vi "UpdateCANData.vi"() -> ()   [LabVIEW 2011]
uses:
  _USB_CAN_T_R_Unit_.ctl
  <vilib>/Utility/file.llb/Write To Spreadsheet File (string).vi
panel:
  in  "sPth_Sel":bool
  out "sv_pth":path
  in  "TSFormat":enum16{"原始值", "实际值"}(ring)
  in  "check2":bool
  in  "rate3":refnum<vi>
  in  "rate2":refnum<vi>
  in  "rate1":refnum<vi>
  in  "errcnt2":refnum<vi>
  in  "Trate2":bool
  in  "Trate1":bool
  in  "Rrate2":bool
  in  "Rrate1":bool
  in  "ForceUpt":bool
  in  "format":enum16{"hex", "dec", "oct", "bin"}(ring)
  in  "ID合并":bool
  in  "SaveCnt":refnum<vi>
  in  "path":refnum<vi>
  in  "rate0":refnum<vi>
  in  "vi ref":refnum<vi>
  in  "highspd":bool
  in  "cancelEvt":refnum<user-event>
  in  "check1":bool
  in  "errcnt1":refnum<vi>
  in  "save":bool
  in  "disp":bool=TRUE
  in  "stop":bool
  in  "savefile":bool
  in  "UseFilter":bool
  in  "Filter":u32[](array[numeric])
  in  "clear":bool
  in  "Enable":bool
  in  "list ref":refnum<vi>
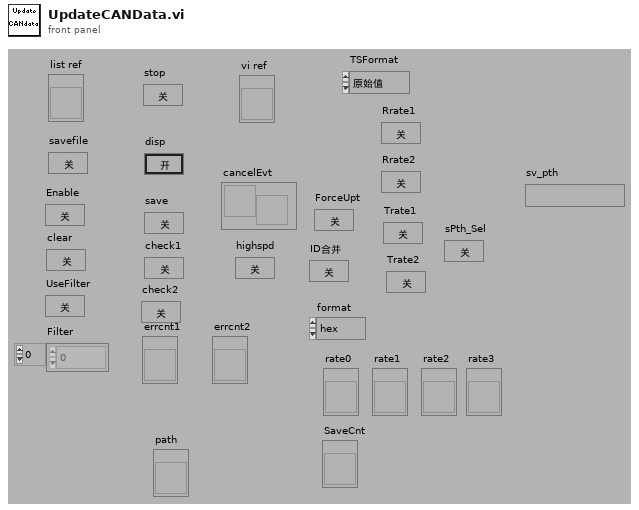
[diagram p1: front panel]
types:
  T1 = typedef "_USB_CAN_T_R_Unit_.ctl" = cluster{"time":timestamp, "channel":u16, "TimeStamp":u32, "tr":enum16{"接收", "发送"}, "id":u32, "Type":enum16{"数据帧", "远程帧"}, "Format":enum16{"标准帧", "扩展帧"}, "len":u8, "data":u8[]}
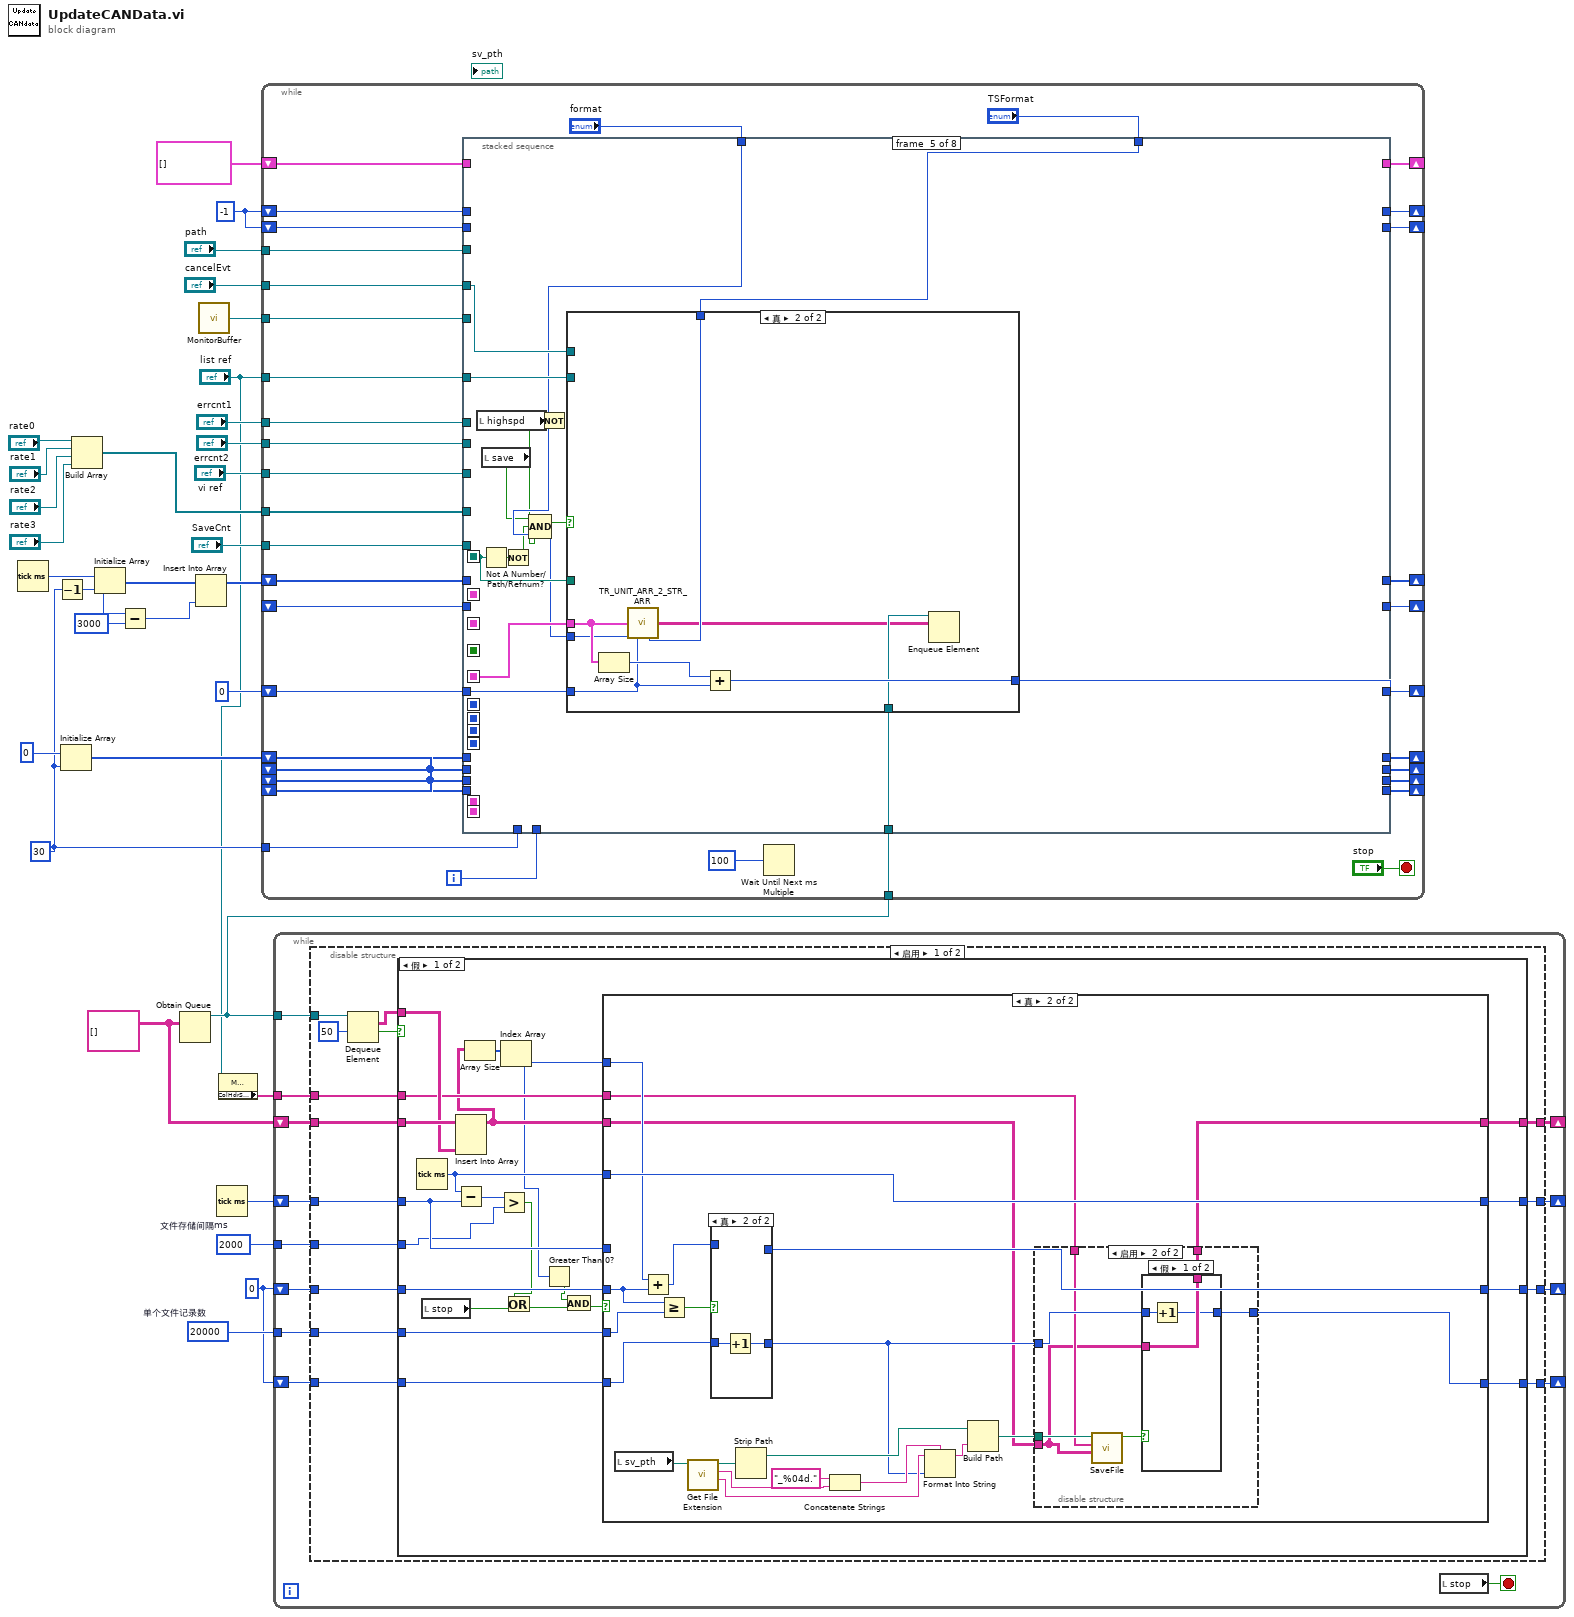
[diagram p0: block diagram]
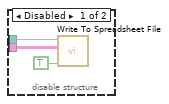
[diagram p3: hidden frame]
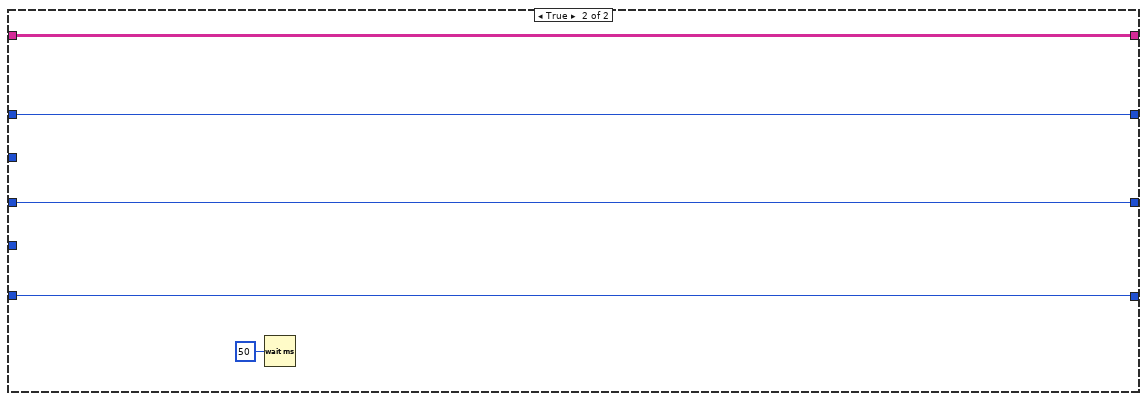
[diagram p6: hidden frame]
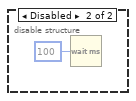
[diagram p7: hidden frame]
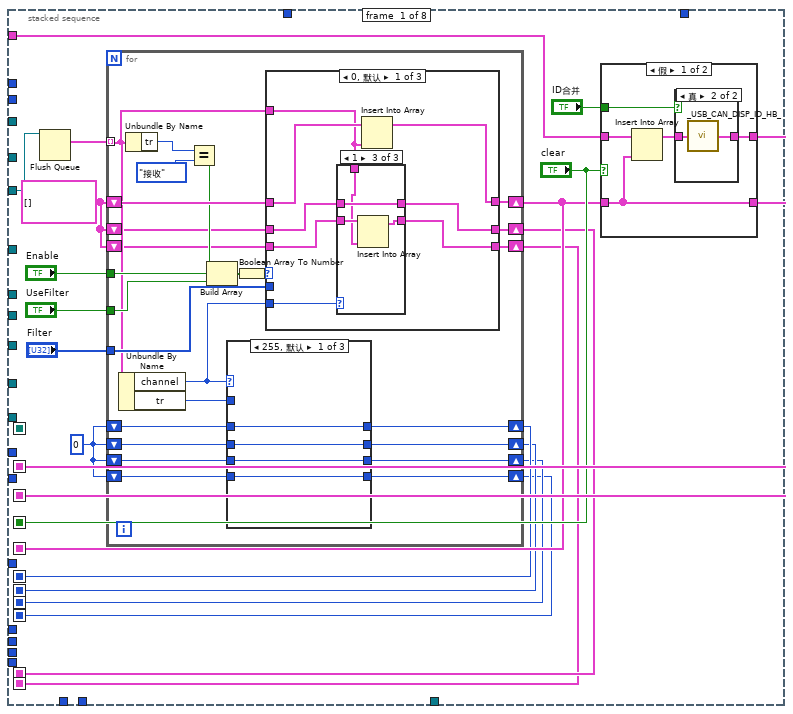
[diagram p8: hidden frame]
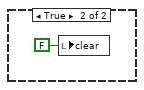
[diagram p10: hidden frame]
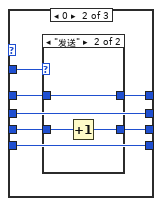
[diagram p11: hidden frame]
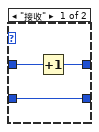
[diagram p12: hidden frame]
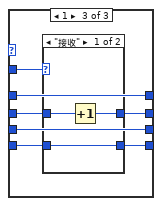
[diagram p13: hidden frame]
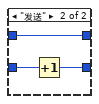
[diagram p14: hidden frame]
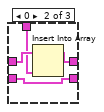
[diagram p16: hidden frame]
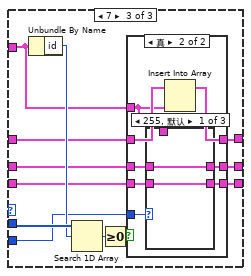
[diagram p18: hidden frame]
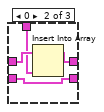
[diagram p20: hidden frame]
diagram:
  w2 = u32 2000  # 文件存储间隔ms
  w3 = 20000  # 单个文件记录数
  w1 = 0
  w8 = string[][] [] ("strTable")
  w25 = 30 ("维数大小")
  w6 = i64 -1 ("U64")
  n1 = Tick Count (ms)() -> (millisecond timer value=w11:u32)
  n2 = Decrement(x=w25) -> (x-1=w24:i32)
  n3 = Initialize Array(0, w25) -> (w17:i32[])
  n4 = Build Array("rate0", "rate1", "rate2", "rate3") -> (w12:refnum<vi>[])
  n5 = Initialize Array(w11, w24) -> (w23:u32[])
  n6 = Subtract(x=w11, y=u32 3000) -> (x-y=w20:u32)
  n7 = Obtain Queue(element data type=w8) -> (queue out=w9:refnum<queue>)  [unwired: 4 in, 2 out]
  n8 = Insert Into Array(array=w23, new element=w20) -> (w22:u32[])  [unwired: 1 in]
  n9 = call "MonitorBuffer.vi"() -> ("USB_CAN_M_BUF"=w32:refnum<queue>)  [unwired: 1 in]
  n10 = Tick Count (ms)() -> (millisecond timer value=w4:u32)
  n11 = property class="MCListbox (严格)"(reference="list ref") -> ("ColHdrString"=w5:string[])  [unwired: 1 in, 2 out]
  n12 = while {
    tunnel: w32 -> [w67]
    shift-right: [w65] -> _
    shift-left: T1[] [] -> [w66]
    tunnel: "list ref" -> [w64]
    shift-right: [w61] -> _
    shift-left: w6 -> [w63]
    tunnel: "errcnt1" -> [w62]
    tunnel: "cancelEvt" -> [w60]
    shift-right: [w58] -> _
    shift-left: 0 -> [w59]
    tunnel: "vi ref" -> [w57]
    shift-right: [w55] -> _
    shift-left: w17 -> [w56]
    tunnel: w25 -> [w53]
    tunnel: w12 -> [w52]
    shift-right: [w50] -> _
    shift-left: w22 -> [w51]
    tunnel: "SaveCnt" -> [w48]
    tunnel: "errcnt2" -> [w46]
    shift-right: [w42] -> _
    shift-left: w17 -> [w45]
    shift-right: [w41] -> _
    shift-left: w17 -> [w44]
    shift-right: [w40] -> _
    shift-left: w17 -> [w43]
    shift-right: [w38] -> _
    shift-left: w6 -> [w39]
    shift-right: [w36] -> _
    shift-left: _ -> [w37]
    tunnel: "path" -> [w34]
    tunnel: w9 -> [w33]
    i -> [w54]
    stop <- "stop" stop-if-true
    n13 = stacked-sequence {
      seq-local: [w85 _ _ _ _ _ _ _] -> [_ _ w300 _ _ w419 _ _]
      seq-local: [w84 _ _ _ _ _ _ _] -> [_ _ w297 _ _ _ _ _]
      seq-local: [_ _ _ w357 _ _ _ _] -> [_ _ _ _ w399 _ _ _]
      seq-local: ["clear" _ _ _ _ _ _ _] -> [_ _ w294 _ _ _ _ _]
      seq-local: [w82 _ _ _ _ _ _ _] -> [_ _ _ _ w396 _ _ _]
      seq-local: [w81 _ _ _ _ _ _ _] -> [_ w228 w292 _ _ _ _ _]
      seq-local: [w80 _ _ _ _ _ _ _] -> [_ w220 w291 _ _ _ _ _]
      seq-local: [w79 _ _ _ _ _ _ _] -> [_ w219 w290 _ _ _ _ _]
      seq-local: [w78 _ _ _ _ _ _ _] -> [_ w218 w289 _ _ _ _ _]
      seq-local: [w77 _ _ _ _ _ _ _] -> [_ _ _ _ _ _ w452 _]
      seq-local: [w76 _ _ _ _ _ _ _] -> [_ _ _ _ _ _ _ w508]
      tunnel: w67 -> [w87 _ _ _ _ _ _ _]
      tunnel: w66 -> [w86 _ _ _ _ _ w455 _]
      tunnel: [_ _ w300 _ _ _ _ _] -> w65
      tunnel: w64 -> [_ _ w299 _ w398 w418 _ _]
      tunnel: w63 -> [_ _ _ _ _ _ w457 _]
      tunnel: w62 -> [_ _ w286 _ _ _ w450 _]
      tunnel: [_ _ _ _ _ _ w458 _] -> w61
      tunnel: w60 -> [_ _ _ _ w397 _ _ _]
      tunnel: w59 -> [_ _ _ _ w395 _ _ _]
      tunnel: [_ _ _ _ w394 _ _ _] -> w58
      tunnel: w57 -> [_ _ w298 _ _ _ _ _]
      tunnel: w56 -> [_ w229 _ _ _ _ _ _]
      tunnel: [_ w227 _ _ _ _ _ _] -> w55
      tunnel: w54 -> [_ w224 _ _ _ _ _ _]
      tunnel: w53 -> [_ w230 _ _ _ _ _ _]
      tunnel: w52 -> [_ w214 _ _ _ _ _ _]
      tunnel: w51 -> [_ w226 _ _ _ _ _ _]
      tunnel: [_ w225 _ _ _ _ _ _] -> w50
      tunnel: w34 -> [_ _ _ w363 _ _ _ _]
      tunnel: w48 -> [_ _ w287 _ _ w417 _ _]
      tunnel: "format" -> [_ _ w296 _ w393 w416 _ _]
      tunnel: w46 -> [_ _ w285 _ _ _ _ w507]
      tunnel: w45 -> [_ w223 _ _ _ _ _ _]
      tunnel: w44 -> [_ w222 _ _ _ _ _ _]
      tunnel: w43 -> [_ w221 _ _ _ _ _ _]
      tunnel: [_ w217 _ _ _ _ _ _] -> w42
      tunnel: [_ w216 _ _ _ _ _ _] -> w41
      tunnel: [_ w215 _ _ _ _ _ _] -> w40
      tunnel: w39 -> [_ _ _ _ _ _ _ w510]
      tunnel: [_ _ _ _ _ _ _ w511] -> w38
      tunnel: w37 -> [_ _ w293 _ _ _ _ _]
      tunnel: [_ _ w295 _ _ _ _ _] -> w36
      tunnel: "TSFormat" -> [_ _ w288 _ w392 _ _ _]
      tunnel: w33 -> [_ _ _ _ w391 _ _ _]
      frame #0 {
        w70 = 0 ("和")
        w69 = T1[] []
        n14 = Flush Queue(queue=w87) -> (remaining elements=w72:T1[])  [unwired: 1 in, 2 out]
        n15 = for {
          tunnel: w72 -> [w111] mode=indexing
          shift-right: [w113] -> w82
          shift-left: w69 -> [w115]
          tunnel: "Enable" -> [w119]
          tunnel: "UseFilter" -> [w118]
          tunnel: "Filter" -> [w114]
          shift-right: [w105] -> w81
          shift-left: w70 -> [w109]
          shift-right: [w104] -> w80
          shift-left: w70 -> [w108]
          shift-right: [w103] -> w79
          shift-left: w70 -> [w107]
          shift-right: [w102] -> w78
          shift-left: w70 -> [w106]
          shift-right: [w99] -> w77
          shift-left: w69 -> [w101]
          shift-right: [w98] -> w76
          shift-left: w69 -> [w100]
          n16 = Unbundle By Name(w111) -> ("channel"=w97:u16, "tr"=w110:enum16{"接收", "发送"})
          n17 = Unbundle By Name(w111) -> ("tr"=w121:enum16{"接收", "发送"})
          n18 = Equal?(x=w121, y=enum16{"接收", "发送"}."接收") -> (x = y?=w112:bool)
          n19 = Build Array(w112, w119, w118) -> (w117:bool[])
          n20 = case shown="255, 默认" w97 {
            tunnel: w110 -> [_ w132 w145]
            tunnel: w109 -> [w125 w130 w144]
            tunnel: w108 -> [w124 w127 w142]
            tunnel: w107 -> [w123 w128 w143]
            tunnel: w106 -> [w122 w131 w141]
            tunnel: [w125 w129 w144] -> w105
            tunnel: [w124 w127 w139] -> w104
            tunnel: [w123 w126 w143] -> w103
            tunnel: [w122 w131 w140] -> w102
            frame 255, Default {
            }
            frame 0 {
              n21 = case shown="\"发送\"" w132 {
                tunnel: w130 -> [w135 w138]
                tunnel: [w134 w138] -> w129
                tunnel: w128 -> [w133 w137]
                tunnel: [w133 w136] -> w126
                frame "接收" {
                  n22 = Increment(x=w135) -> (x+1=w134:i32)
                }
                frame "发送" {
                  n23 = Increment(x=w137) -> (x+1=w136:i32)
                }
              }
            }
            frame 1 {
              n24 = case shown="\"接收\"" w145 {
                tunnel: w142 -> [w148 w149]
                tunnel: w141 -> [w146 w151]
                tunnel: [w146 w150] -> w140
                tunnel: [w147 w149] -> w139
                frame "接收" {
                  n25 = Increment(x=w148) -> (x+1=w147:i32)
                }
                frame "发送" {
                  n26 = Increment(x=w151) -> (x+1=w150:i32)
                }
              }
            }
          }
          n27 = Boolean Array To Number(Boolean array=w117) -> (number=w116:u32)
          n28 = case shown="0, 默认" w116 {
            tunnel: w115 -> [w158 w172 w180]
            tunnel: w111 -> [w157 _ w179]
            tunnel: w114 -> [_ _ w184]
            tunnel: [w159 w172 w178] -> w113
            tunnel: w101 -> [w155 w171 w176]
            tunnel: w100 -> [w154 w170 w175]
            tunnel: [w153 w171 w174] -> w99
            tunnel: [w152 w170 w173] -> w98
            tunnel: w97 -> [w156 _ w177]
            frame 0, Default {
              n29 = case shown="1" w156 {
                tunnel: w155 -> [w161 w165 w169]
                tunnel: w154 -> [w160 w163 w167]
                tunnel: [w161 w164 w169] -> w153
                tunnel: [w160 w163 w168] -> w152
                tunnel: w157 -> [_ w162 w166]
                frame 255, Default {
                }
                frame 0 {
                  n30 = Insert Into Array(array=w165, new element=w162) -> (w164:T1[])  [unwired: 1 in]
                }
                frame 1 {
                  n31 = Insert Into Array(array=w167, new element=w166) -> (w168:T1[])  [unwired: 1 in]
                }
              }
              n32 = Insert Into Array(array=w158, new element=w157) -> (w159:T1[])  [unwired: 1 in]
            }
            frame 1, 5 {
            }
            frame 7 {
              n33 = Unbundle By Name(w179) -> ("id"=w183:u32)
              n34 = Search 1D Array(1D array=w184, element=w183) -> (index of element=w182:i32)  [unwired: 1 in]
              n35 = Greater Or Equal To 0?(x=w182) -> (x >= 0?=w181:bool)
              n36 = case shown="真" w181 {
                tunnel: w180 -> [w187 w195]
                tunnel: w179 -> [_ w188]
                tunnel: [w187 w194] -> w178
                tunnel: w177 -> [_ w193]
                tunnel: w176 -> [w186 w192]
                tunnel: w175 -> [w185 w191]
                tunnel: [w186 w190] -> w174
                tunnel: [w185 w189] -> w173
                frame False {
                }
                frame True {
                  n37 = case shown="255, 默认" w193 {
                    tunnel: w192 -> [w197 w201 w205]
                    tunnel: w191 -> [w196 w199 w203]
                    tunnel: [w197 w200 w205] -> w190
                    tunnel: [w196 w199 w204] -> w189
                    tunnel: w188 -> [_ w198 w202]
                    frame 255, Default {
                    }
                    frame 0 {
                      n38 = Insert Into Array(array=w201, new element=w198) -> (w200:T1[])  [unwired: 1 in]
                    }
                    frame 1 {
                      n39 = Insert Into Array(array=w203, new element=w202) -> (w204:T1[])  [unwired: 1 in]
                    }
                  }
                  n40 = Insert Into Array(array=w195, new element=w188) -> (w194:T1[])  [unwired: 1 in]
                }
              }
            }
          }
        }
        n41 = case shown="假" "clear" {
          tunnel: w82 -> [w92 _]
          tunnel: w86 -> [w91 _]
          tunnel: [w88 _] -> w85
          tunnel: [w92 _] -> w84
          tunnel: "ID合并" -> [w90 _]
          frame False {
            n42 = Insert Into Array(array=w91, new element=w92) -> (w89:T1[])  [unwired: 1 in]
            n43 = case shown="真" w90 {
              tunnel: w89 -> [w93 w95]
              tunnel: [w93 w94] -> w88
              frame False {
              }
              frame True {
                n44 = call "_USB_CAN_DISP_ID_HB_.vi"("Arr In"=w95) -> ("Arr Out"=w94:T1[])
              }
            }
          }
          frame True {
            n45 = local write "clear"(FALSE ("clear")) -> ()
          }
        }
      }
      frame #1 {
        n46 = Tick Count (ms)() -> (millisecond timer value=w213:u32)
        n47 = Quotient & Remainder(x=w224, y=w230) -> (x-y*floor(x/y)=w210:i32)  [unwired: 1 out]
        n48 = Replace Array Subset(array=w229, new element=w228, index=w210) -> (w227:i32[])
        n49 = Replace Array Subset(array=w223, new element=w220, index=w210) -> (w217:i32[])
        n50 = Replace Array Subset(array=w222, new element=w219, index=w210) -> (w216:i32[])
        n51 = Replace Array Subset(array=w221, new element=w218, index=w210) -> (w215:i32[])
        n52 = Replace Array Subset(array=w226, new element=w213, index=w210) -> (w225:u32[])
        n53 = Quotient & Remainder(x=w224, y=5) -> (x-y*floor(x/y)=w211:i32)  [unwired: 1 out]
        n54 = case shown="0" w211 {
          tunnel: w227 -> [_ w248]
          tunnel: w225 -> [_ w245]
          tunnel: w217 -> [_ w238]
          tunnel: w216 -> [_ w237]
          tunnel: w215 -> [_ w236]
          tunnel: w214 -> [_ w244]
          tunnel: "Rrate1" -> [_ w234]
          tunnel: "Rrate2" -> [_ w233]
          tunnel: "Trate1" -> [_ w232]
          tunnel: "Trate2" -> [_ w231]
          frame -1, Default {
          }
          frame 0 {
            w235 = 1000.0 ("y")
            n55 = Array Max & Min(array=w245) -> (max value=w247:u32, min value=w246:u32)  [unwired: 2 out]
            n56 = Subtract(x=w247, y=w246) -> (x-y=w239:u32)
            n57 = Index Array(array=w244) -> (element #1=w243:refnum<vi>, element #2=w242:refnum<vi>, element #3=w241:refnum<vi>, element #4=w240:refnum<vi>)  [unwired: 4 in]
            n58 = case shown="真" w234 {
              tunnel: w248 -> [_ w276]
              tunnel: w243 -> [_ w272]
              tunnel: w239 -> [_ w271]
              tunnel: w235 -> [_ w270]
              frame False {
              }
              frame True {
                n59 = Add Array Elements(numeric array=w276) -> (sum=w275:i32)
                n60 = Divide(x=w275, y=w271) -> (x/y=w274:dbl)
                n61 = Multiply(x=w274, y=w270) -> (x*y=w273:dbl)
                n62 = property class="DigNum (严格)"(reference=w272, "Value"=w273) -> ()  [unwired: 1 in, 2 out]
              }
            }
            n63 = case shown="真" w233 {
              tunnel: w242 -> [_ w266]
              tunnel: w239 -> [_ w265]
              tunnel: w238 -> [_ w264]
              tunnel: w235 -> [_ w263]
              frame False {
              }
              frame True {
                n64 = Add Array Elements(numeric array=w264) -> (sum=w267:i32)
                n65 = Divide(x=w267, y=w265) -> (x/y=w268:dbl)
                n66 = Multiply(x=w268, y=w263) -> (x*y=w269:dbl)
                n67 = property class="DigNum (严格)"(reference=w266, "Value"=w269) -> ()  [unwired: 1 in, 2 out]
              }
            }
            n68 = case shown="真" w232 {
              tunnel: w241 -> [_ w259]
              tunnel: w239 -> [_ w258]
              tunnel: w237 -> [_ w257]
              tunnel: w235 -> [_ w256]
              frame False {
              }
              frame True {
                n69 = Add Array Elements(numeric array=w257) -> (sum=w262:i32)
                n70 = Divide(x=w262, y=w258) -> (x/y=w261:dbl)
                n71 = Multiply(x=w261, y=w256) -> (x*y=w260:dbl)
                n72 = property class="DigNum (严格)"(reference=w259, "Value"=w260) -> ()  [unwired: 1 in, 2 out]
              }
            }
            n73 = case shown="真" w231 {
              tunnel: w240 -> [_ w252]
              tunnel: w239 -> [_ w251]
              tunnel: w236 -> [_ w250]
              tunnel: w235 -> [_ w249]
              frame False {
              }
              frame True {
                n74 = Add Array Elements(numeric array=w250) -> (sum=w253:i32)
                n75 = Divide(x=w253, y=w251) -> (x/y=w254:dbl)
                n76 = Multiply(x=w254, y=w249) -> (x*y=w255:dbl)
                n77 = property class="DigNum (严格)"(reference=w252, "Value"=w255) -> ()  [unwired: 1 in, 2 out]
              }
            }
          }
        }
      }
      frame #2 {
        n78 = Not A Number/Path/Refnum?(number/path/refnum=w299) -> (NaN/Path/Refnum?=w284:bool)
        n79 = Empty Array?(array=w297) -> (empty?=w282:bool)
        n80 = Compound Arithmetic op=AND("disp", invert w284, invert w282, invert "highspd") -> (w281:bool)
        n81 = Compound Arithmetic op=ADD(w292, w291, w290, w289) -> (w278:i32)
        n82 = Compound Arithmetic op=OR("ForceUpt", w281, w294) -> (w280:bool)
        n83 = case shown="真" w280 {
          tunnel: w299 -> [_ w321]
          tunnel: w300 -> [_ w322]
          tunnel: w298 -> [_ w320]
          tunnel: w297 -> [_ w319]
          tunnel: w296 -> [_ w318]
          tunnel: w293 -> [w301 w307]
          tunnel: [w301 w317] -> w295
          tunnel: "ForceUpt" -> [_ w316]
          tunnel: w294 -> [_ w315]
          tunnel: w278 -> [_ w313]
          tunnel: w288 -> [_ w305]
          tunnel: w287 -> [_ _]
          tunnel: w286 -> [_ w303]
          tunnel: w285 -> [_ w302]
          frame False {
          }
          frame True {
            n84 = Tick Count (ms)() -> (millisecond timer value=w314:u32)
            n85 = Greater?(x=w313, y=0) -> (0:w306:bool)
            n86 = Subtract(x=w314, y=w307) -> (x-y=w311:u32)
            n87 = Greater?(x=w311, y=u32 300) -> (0:w309:bool)
            n88 = And(x=w309, y=w306) -> (x .and. y?=w308:bool)
            n89 = Compound Arithmetic op=OR(w316, w315, w308, w306) -> (w304:bool)
            n90 = case shown="真" w304 {
              tunnel: w322 -> [_ w332]
              tunnel: w321 -> [_ w331]
              tunnel: w320 -> [_ w330]
              tunnel: w319 -> [_ w329]
              tunnel: w318 -> [_ w328]
              tunnel: [w323 w327] -> w317
              tunnel: w314 -> [_ w327]
              tunnel: w307 -> [w323 _]
              tunnel: w305 -> [_ w326]
              tunnel: w303 -> [_ w325]
              tunnel: w302 -> [_ w324]
              frame False {
              }
              frame True {
                n91 = stacked-sequence {
                  tunnel: w332 -> [_ w349 _]
                  tunnel: w331 -> [_ w351 _]
                  tunnel: w330 -> [w333 _ w352]
                  tunnel: w329 -> [_ _ _]
                  tunnel: w328 -> [_ w350 _]
                  tunnel: w326 -> [_ w341 _]
                  tunnel: w325 -> [_ _ _]
                  tunnel: w324 -> [_ _ _]
                  frame #0 {
                    n92 = property class="VI"(reference=w333) -> (error out=w334:errorcluster, "Panel"=w336:refnum<vi>)  [unwired: 1 in, 1 out]
                    n93 = property class="Pnl"(reference=w336, error in=w334, "DeferPanUpdts"=TRUE ("延迟前面板更新")) -> ()  [unwired: 2 out]
                  }
                  frame #1 {
                    n94 = Array Size(array=w349) -> (size(s)=w347:i32)
                    n95 = Subtract(x=w347, y=200) -> (x-y=w343:i32)
                    n96 = Less Than 0?(x=w343) -> (x < 0?=w345:bool)
                    n97 = Select(t=0, s=w345, f=w343) -> (s? t:f=w342:i32)
                    n98 = Array Subset(array=w349, index=w342) -> (w348:T1[])  [unwired: 1 in]
                    n99 = call "TR_UNIT_ARR_2_STR_ARR.vi"("offset"=w342, "TR_Unit_Arr"=w348, "format"=w350, "TSFormat"=w341) -> ("smb"=w338:i32[], "strTable"=w339:string[][])  [unwired: 10 in]
                    n100 = property class="MCListbox (严格)"(reference=w351, "ItemNames"=w339, "ItemSyms"=w338) -> (reference out=w340:refnum<vi>)  [unwired: 1 in, 1 out]
                    n101 = call "DispLastRow(MList).vi"("显示尾行"=TRUE, "MCListbox引用句柄"=w340) -> ()  [unwired: 8 in, 2 out]
                  }
                  frame #2 {
                    n102 = property class="VI"(reference=w352) -> (error out=w353:errorcluster, "Panel"=w355:refnum<vi>)  [unwired: 1 in, 1 out]
                    n103 = property class="Pnl"(reference=w355, error in=w353, "DeferPanUpdts"=FALSE ("延迟前面板更新")) -> ()  [unwired: 2 out]
                  }
                }
              }
            }
          }
        }
      }
      frame #3 {
        n104 = local read "highspd"() -> (w362:bool)
        n105 = local read "sv_pth"() -> (w358:path)
        n106 = Not(x=w362) -> (.not. x?=w359:bool)
        n107 = And(x="save", y=w359) -> (x .and. y?=w360:bool)
        n108 = case shown="真" w360 {
          tunnel: w358 -> [w364 w369]
          tunnel: [w364 w372] -> w357
          tunnel: w363 -> [_ w371]
          tunnel: [_ w370] -> w356
          frame False {
          }
          frame True {
            n109 = Not A Number/Path/Refnum?(number/path/refnum=w369) -> (NaN/Path/Refnum?=w368:bool)
            n110 = Empty String/Path?(string/path=w369) -> (empty?=w367:bool)
            n111 = Compound Arithmetic op=OR(w368, w367, "sPth_Sel") -> (w366:bool)
            n112 = case shown="真" w366 {
              tunnel: w369 -> [w373 _]
              tunnel: [w373 w376] -> w372
              frame False {
              }
              frame True {
                n113 = call "文件对话框"("prompt"="File Save As", "pattern (all files)"="*.xls", "pattern label"="Excel File") -> ("selected path"=w377:path, "cancelled"=w379:bool, "error out"=w381:errorcluster)  [unwired: 9 in, 1 out]
                n114 = Unbundle By Name(w381) -> ("status"=w380:bool)
                n115 = local write "sPth_Sel"(FALSE ("sPth_Sel")) -> ()
                n116 = Or(x=w379, y=w380) -> (x .or. y?=w378:bool)
                n117 = Select(t=path "", s=w378, f=w377) -> (s? t:f=w376:path)
              }
            }
            n118 = property class="Path"(reference=w371, "Value"=w372) -> (error out=w370:errorcluster)  [unwired: 1 in, 1 out]
          }
        }
        n119 = call <vilib>:"Simple Error Handler.vi"("error in (no error)"=w356) -> ()  [unwired: 4 in, 5 out]
        n120 = local write "sv_pth"(w357) -> ()
      }
      frame #4 {
        n121 = local read "highspd"() -> (w386:bool)
        n122 = Not A Number/Path/Refnum?(number/path/refnum=w399) -> (NaN/Path/Refnum?=w390:bool)
        n123 = local read "save"() -> (w389:bool)
        n124 = Not(x=w390) -> (.not. x?=w388:bool)
        n125 = Not(x=w386) -> (.not. x?=w385:bool)
        n126 = Compound Arithmetic op=AND(w389, w388, w385) -> (w387:bool)
        n127 = case shown="真" w387 {
          tunnel: w396 -> [_ w414]
          tunnel: w399 -> [_ _]
          tunnel: w398 -> [_ _]
          tunnel: w397 -> [w402 _]
          tunnel: w395 -> [w400 w411]
          tunnel: [w400 w413] -> w394
          tunnel: w393 -> [_ w410]
          tunnel: w392 -> [_ w409]
          tunnel: w391 -> [_ w408]
          frame False {
            n128 = local read "save"() -> (w401:bool)
            n129 = case shown="真" w401 {
              tunnel: w402 -> [_ w405]
              frame False {
              }
              frame True {
                n130 = Generate User Event(user event=w405, event data cluster=FALSE ("事件数据")) -> (error out=w403:errorcluster)  [unwired: 1 in, 1 out]
                n131 = local write "save"(FALSE ("save")) -> ()
                n132 = call <vilib>:"Simple Error Handler.vi"("error in (no error)"=w403) -> ()  [unwired: 4 in, 5 out]
              }
            }
          }
          frame True {
            n133 = Array Size(array=w414) -> (size(s)=w412:i32)
            n134 = call "TR_UNIT_ARR_2_STR_ARR.vi"("offset"=w411, "TR_Unit_Arr"=w414, "format"=w410, "TSFormat"=w409) -> ("strTable"=w407:string[][])  [unwired: 10 in, 1 out]
            n135 = Add(x=w412, y=w411) -> (x+y=w413:i32)
            n136 = Enqueue Element(queue=w408, element=w407) -> ()  [unwired: 2 in, 3 out]
          }
        }
      }
      frame #5 {
        n137 = case shown="真" "savefile" {
          tunnel: w419 -> [_ w424]
          tunnel: w418 -> [_ w423]
          tunnel: w417 -> [_ w421]
          tunnel: w416 -> [_ w420]
          frame False {
          }
          frame True {
            n138 = local write "savefile"(FALSE ("savefile")) -> ()
            n139 = call "文件对话框2"("prompt"="File Save As", "pattern (all files)"="*.xls", "pattern label"="Excel File") -> ("selected path"=w425:path, "exists"=w429:bool, "cancelled"=w430:bool, "error out"=w432:errorcluster)  [unwired: 9 in]
            n140 = Unbundle By Name(w432) -> ("status"=w431:bool)
            n141 = Not And(1:w431, 2:w430) -> (0:w427:bool)
            n142 = case shown="真" w429 {
              tunnel: [TRUE ("T button?") w447] -> w428
              frame False {
              }
              frame True {
                n143 = Two Button Dialog(message="所选文件已存在，是否替换？" ("消息"), 2:"替换" ("T按钮名称（“确定”）")) -> (T button?=w447:bool)  [unwired: 1 in]
              }
            }
            n144 = And(x=w428, y=w427) -> (x .and. y?=w426:bool)
            n145 = case shown="真" w426 {
              tunnel: w425 -> [_ w444]
              tunnel: w424 -> [_ w439]
              tunnel: w423 -> [_ w445]
              tunnel: [_ w438] -> w422
              tunnel: w420 -> [_ w437]
              frame False {
              }
              frame True {
                n146 = property class="MCListbox (严格)"(reference=w445) -> ("ColHdrString"=w442:string[])  [unwired: 1 in, 2 out]
                n147 = call "TR_UNIT_ARR_2_STR_ARR.vi"("TR_Unit_Arr"=w439, "format"=w437) -> ("strTable"=w440:string[][])  [unwired: 12 in, 1 out]
                n148 = Insert Into Array(array=w440, index (row)=0 ("索引 (行)"), new element=w442) -> (w441:string[][])  [unwired: 1 in]
                n149 = call-poly <vilib>:"Write To Spreadsheet File.vi"("2D data"=w441, "file path (dialog if empty)"=w444) -> ()  [unwired: 6 in, 1 out]
                n150 = Array Size(array=w439) -> (size(s)=w438:i32)
              }
            }
            n151 = property class="DigNum (严格)"(reference=w421, "Value"=w422) -> ()  [unwired: 1 in, 2 out]
          }
        }
      }
      frame #6 {
        n152 = Array Size(array=w455) -> (size(s)=w454:i32)
        n153 = case shown="真" "check1" {
          tunnel: w452 -> [_ w470]
          tunnel: [i64 -1 ("U64") w463] -> w458
          tunnel: w457 -> [_ w468]
          tunnel: w450 -> [w462 w471]
          frame False {
            n154 = property class="DigNum (严格)"(reference=w462, "Value"=0 ("值")) -> ()  [unwired: 1 in, 2 out]
          }
          frame True {
            n155 = for {
              tunnel: w470 -> [w491] mode=indexing
              shift-right: [w489] -> w463
              shift-left: w468 -> [w488]
              tunnel: [w487] -> w469
              tunnel: [w486] -> w467
              shift-right: [w483] -> w464
              shift-left: i64[] [] -> [w484]
              n156 = Unbundle By Name(w491) -> ("tr"=w485:enum16{"接收", "发送"}, "id"=w486:u32, "data"=w490:u8[], "time"=w487:timestamp)
              n157 = case shown="\"接收\", 默认" w485 {
                tunnel: w490 -> [w499 _]
                tunnel: [w492 w506] -> w489
                tunnel: w488 -> [w493 w506]
                tunnel: w484 -> [w495 w505]
                tunnel: [w494 w505] -> w483
                frame "接收", Default {
                  n158 = call "U8_Arr_To_I64.vi"("data"=w499) -> ("I64"=w492:i64)
                  n159 = Subtract(x=w492, y=w493) -> (x-y=w498:i64)
                  n160 = Equal?(x=i64 1, y=w498) -> (x = y?=w496:bool)
                  n161 = case shown="假" w496 {
                    tunnel: w495 -> [w503 w504]
                    tunnel: [w502 w504] -> w494
                    tunnel: w493 -> [w501 _]
                    tunnel: w492 -> [w500 _]
                    frame False {
                      n162 = Insert Into Array(array=w503, new element #1=w501, new element #2=w500) -> (w502:i64[])  [unwired: 1 in]
                    }
                    frame True {
                    }
                  }
                }
                frame "发送" {
                }
              }
            }
            n163 = Empty Array?(array=w464) -> (empty?=w465:bool)
            n164 = case shown="假" w465 {
              tunnel: w471 -> [w482 _]
              tunnel: w469 -> [w479 _]
              tunnel: w467 -> [w478 _]
              tunnel: w464 -> [w475 _]
              frame False {
                n165 = property class="DigNum (严格)"(reference=w482) -> (reference out=w481:refnum<vi>, error out=w480:errorcluster, "Value"=w477:i32)  [unwired: 1 in]
                n166 = Array Size(array=w475) -> (size(s)=w474:i32)
                n167 = Divide(x=w474, y=2) -> (x/y=w472:dbl)
                n168 = Add(x=w477, y=w472) -> (x+y=w476:dbl)
                n169 = call "_USB_CAN_DEBUG_LOG_OUT_.vi"("id"=w478, "Edata"=w475, "TIME"=w479) -> ()  [unwired: 9 in]
                n170 = property class="DigNum (严格)"(reference=w481, error in=w480, "Value"=w476) -> ()  [unwired: 2 out]
              }
              frame True {
              }
            }
          }
        }
        n171 = Greater?(x=w454, y=99999) -> (0:w451:bool)
        n172 = case shown="真" w451 {
          frame False {
          }
          frame True {
            n173 = local write "clear"(TRUE ("clear")) -> ()
          }
        }
      }
      frame #7 {
        n174 = case shown="真" "check2" {
          tunnel: w508 -> [_ w522]
          tunnel: [i64 -1 ("U64") w515] -> w511
          tunnel: w510 -> [_ w520]
          tunnel: w507 -> [w514 w523]
          frame False {
            n175 = property class="DigNum (严格)"(reference=w514, "Value"=0 ("值")) -> ()  [unwired: 1 in, 2 out]
          }
          frame True {
            n176 = for {
              tunnel: w522 -> [w543] mode=indexing
              shift-right: [w541] -> w515
              shift-left: w520 -> [w540]
              tunnel: [w539] -> w521
              tunnel: [w538] -> w519
              shift-right: [w535] -> w516
              shift-left: i64[] [] -> [w536]
              n177 = Unbundle By Name(w543) -> ("tr"=w537:enum16{"接收", "发送"}, "id"=w538:u32, "data"=w542:u8[], "time"=w539:timestamp)
              n178 = case shown="\"接收\", 默认" w537 {
                tunnel: w542 -> [w551 _]
                tunnel: [w544 w558] -> w541
                tunnel: w540 -> [w545 w558]
                tunnel: w536 -> [w547 w557]
                tunnel: [w546 w557] -> w535
                frame "接收", Default {
                  n179 = call "U8_Arr_To_I64.vi"("data"=w551) -> ("I64"=w544:i64)
                  n180 = Subtract(x=w544, y=w545) -> (x-y=w550:i64)
                  n181 = Equal?(x=i64 1, y=w550) -> (x = y?=w548:bool)
                  n182 = case shown="假" w548 {
                    tunnel: w547 -> [w555 w556]
                    tunnel: [w554 w556] -> w546
                    tunnel: w545 -> [w553 _]
                    tunnel: w544 -> [w552 _]
                    frame False {
                      n183 = Insert Into Array(array=w555, new element #1=w553, new element #2=w552) -> (w554:i64[])  [unwired: 1 in]
                    }
                    frame True {
                    }
                  }
                }
                frame "发送" {
                }
              }
            }
            n184 = Empty Array?(array=w516) -> (empty?=w517:bool)
            n185 = case shown="假" w517 {
              tunnel: w523 -> [w534 _]
              tunnel: w521 -> [w531 _]
              tunnel: w519 -> [w530 _]
              tunnel: w516 -> [w527 _]
              frame False {
                n186 = property class="DigNum (严格)"(reference=w534) -> (reference out=w533:refnum<vi>, error out=w532:errorcluster, "Value"=w529:i32)  [unwired: 1 in]
                n187 = Array Size(array=w527) -> (size(s)=w526:i32)
                n188 = Divide(x=w526, y=2) -> (x/y=w524:dbl)
                n189 = Add(x=w529, y=w524) -> (x+y=w528:dbl)
                n190 = call "_USB_CAN_DEBUG_LOG_OUT_.vi"("id"=w530, "Edata"=w527, "TIME"=w531) -> ()  [unwired: 9 in]
                n191 = property class="DigNum (严格)"(reference=w533, error in=w532, "Value"=w528) -> ()  [unwired: 2 out]
              }
              frame True {
              }
            }
          }
        }
      }
    }
    n192 = Wait Until Next ms Multiple(millisecond multiple=u32 100 ("毫秒倍数")) -> ()  [unwired: 1 out]
  }
  n193 = while {
    tunnel: w9 -> [w570]
    shift-right: [w568] -> _
    shift-left: w8 -> [w569]
    tunnel: w5 -> [w567]
    shift-right: [w565] -> _
    shift-left: w4 -> [w566]
    shift-right: [w563] -> _
    shift-left: w1 -> [w564]
    tunnel: w3 -> [w562]
    tunnel: w2 -> [w561]
    shift-right: [w559] -> _
    shift-left: w1 -> [w560]
    stop <- w571 stop-if-true
    n194 = disable-structure shown="启用" {
      disable-tunnel: w570 -> [w586 _]
      disable-tunnel: w569 -> [w582 _]
      disable-tunnel: [w581 _] -> w568
      disable-tunnel: w567 -> [w580 _]
      disable-tunnel: w566 -> [w579 _]
      disable-tunnel: [w578 _] -> w565
      disable-tunnel: w564 -> [w577 _]
      disable-tunnel: [w576 _] -> w563
      disable-tunnel: w562 -> [w575 _]
      disable-tunnel: w561 -> [w574 _]
      disable-tunnel: w560 -> [w573 _]
      disable-tunnel: [w572 _] -> w559
      frame Enabled {
        n195 = Dequeue Element(queue=w586, timeout in ms (-1)=50 ("超时毫秒(-1)")) -> (element=w583:string[][], timed out?=w584:bool)  [unwired: 1 in, 2 out]
        n196 = case shown="假" w584 {
          tunnel: w583 -> [w607 _]
          tunnel: w582 -> [w608 w657]
          tunnel: [w599 w657] -> w581
          tunnel: w580 -> [w602 _]
          tunnel: w579 -> [w604 w656]
          tunnel: [w603 w656] -> w578
          tunnel: w577 -> [w601 w655]
          tunnel: [w600 w655] -> w576
          tunnel: w575 -> [w596 _]
          tunnel: w574 -> [w595 _]
          tunnel: w573 -> [w588 w654]
          tunnel: [w587 w654] -> w572
          frame False {
            n197 = Tick Count (ms)() -> (millisecond timer value=w605:u32)
            n198 = local read "stop"() -> (w597:bool)
            n199 = Insert Into Array(array=w608, new element=w607) -> (w593:string[][])  [unwired: 2 in]
            n200 = Subtract(x=w605, y=w604) -> (x-y=w606:u32)
            n201 = Array Size(array=w593) -> (size(s)=w594:i32[])
            n202 = Greater?(x=w606, y=w595) -> (0:w598:bool)
            n203 = Index Array(array=w594) -> (element=w589:i32)  [unwired: 1 in]
            n204 = Or(x=w598, y=w597) -> (x .or. y?=w592:bool)
            n205 = Greater Than 0?(x=w589) -> (x > 0?=w590:bool)
            n206 = And(x=w590, y=w592) -> (x .and. y?=w591:bool)
            n207 = case shown="真" w591 {
              tunnel: w605 -> [_ w634]
              tunnel: w604 -> [w612 _]
              tunnel: [w612 w634] -> w603
              tunnel: w602 -> [_ w613]
              tunnel: w601 -> [w611 w622]
              tunnel: [w611 w620] -> w600
              tunnel: w593 -> [w610 w614]
              tunnel: [w610 w618] -> w599
              tunnel: w596 -> [_ w628]
              tunnel: w589 -> [_ w629]
              tunnel: w588 -> [w609 w615]
              tunnel: [w609 w617] -> w587
              frame False {
              }
              frame True {
                n208 = local read "sv_pth"() -> (w630:path)
                n209 = Add(x=w629, y=w622) -> (x+y=w621:i32)
                n210 = Greater Or Equal?(x=w622, y=w628) -> (x >= y?=w619:bool)
                n211 = call <vilib>:"Get File Extension.vi"("file"=w630) -> ("filename without extension"=w627:string, "lowercase file extension"=w632:string, "dup file"=w631:path)  [unwired: 7 in, 1 out]
                n212 = case shown="真" w619 {
                  tunnel: w615 -> [w649 w652]
                  tunnel: [w649 w651] -> w616
                  tunnel: w621 -> [w650 _]
                  tunnel: [w650 _] -> w620
                  frame False {
                  }
                  frame True {
                    n213 = Increment(x=w652) -> (x+1=w651:i32)
                  }
                }
                n214 = Strip Path(path=w631) -> (stripped path=w625:path)  [unwired: 1 out]
                n215 = Concatenate Strings("_%04d." ("字符串"), w632) -> (w626:string)
                n216 = Format Into String(format string=w626, initial string=w627, w616) -> (resulting string=w624:string)  [unwired: 1 in, 1 out]
                n217 = Build Path(base path=w625, name or relative path=w624) -> (appended path=w623:path)
                n218 = disable-structure shown="启用" {
                  disable-tunnel: w614 -> [w637 w639]
                  disable-tunnel: w623 -> [w635 w641]
                  disable-tunnel: [_ w644] -> w618
                  disable-tunnel: w616 -> [_ w643]
                  disable-tunnel: [_ w642] -> w617
                  disable-tunnel: w613 -> [_ w640]
                  frame Disabled {
                    n219 = call-poly <vilib>:"Write To Spreadsheet File.vi"("append to file? (new file:F)"=TRUE, "2D data"=w637, "file path (dialog if empty)"=w635) -> ()  [unwired: 5 in, 1 out]
                  }
                  frame Enabled {
                    n220 = call "SaveFile.vi"("数据"=w639, "文件头"=w640, "文件路径"=w641) -> ("Success"=w638:bool)  [unwired: 8 in]
                    n221 = case shown="假" w638 {
                      tunnel: w639 -> [w647 _]
                      tunnel: [w647 _] -> w644
                      tunnel: w643 -> [w646 w648]
                      tunnel: [w645 w648] -> w642
                      frame False {
                        n222 = Increment(x=w646) -> (x+1=w645:i32)
                      }
                      frame True {
                      }
                    }
                  }
                }
              }
            }
          }
          frame True {
            n223 = Wait (ms)(milliseconds to wait=u32 50 ("等待时间（毫秒）")) -> ()  [unwired: 1 out]
          }
        }
      }
      frame Disabled {
        n224 = Wait (ms)(milliseconds to wait=u32 100 ("等待时间（毫秒）")) -> ()  [unwired: 1 out]
      }
    }
    n225 = local read "stop"() -> (w571:bool)
  }
